vi "new Resource Name Filter.vi"(10 "Resource Name":string) -> (2 "resource name filter out":refnum<class "Filter.lvclass">)   [LabVIEW 2016, in "Resource Name Filter.lvclass"]
uses:
  Resource Name Filter.lvclass
  Filter Parent/Filter.lvclass
  C:/github/VeriStand-FPGA-Resource-Manager/Source/Client/Test CD/FPGA RM Test Client/Source/System Explorer/Filters/Filter Parent/Filter.lvclass
  Resource Name Filter.lvclass/Resource Name Filter.ctl
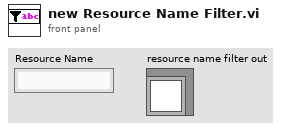
[diagram p1: front panel]
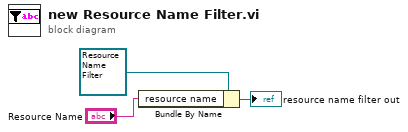
[diagram p0: block diagram]
diagram:
  n1 = Bundle By Name(cluster=refnum<class "Resource Name Filter.lvclass"> refnum ("Resource Name Filter out"), "resource name"="Resource Name") -> (→"resource name filter out":refnum<class "Resource Name Filter.lvclass">)
